vi "decodeModbusMessage.vi"(8 "error in (no error)":errorcluster, 10 "Enc_values_in":T1, 11 "VISA resource name":refnum<visa-resource-name>) -> (0 "error out":errorcluster, 2 "Enc_values_out 2":T1, 3 "VISA Refnum out":refnum<visa-resource-name>)   [LabVIEW 2026]
uses:
  Control/Ctr_Enc_Values.ctl
  Control/Ctrl_Motores_Valores.ctl
  Control/Ctrl_Errores.ctl
  Control/Ctrl_Modbus64.ctl
  Control/Ctrl_Datos6Motores.ctl
  Control/Ctrl_Modbus13.ctl
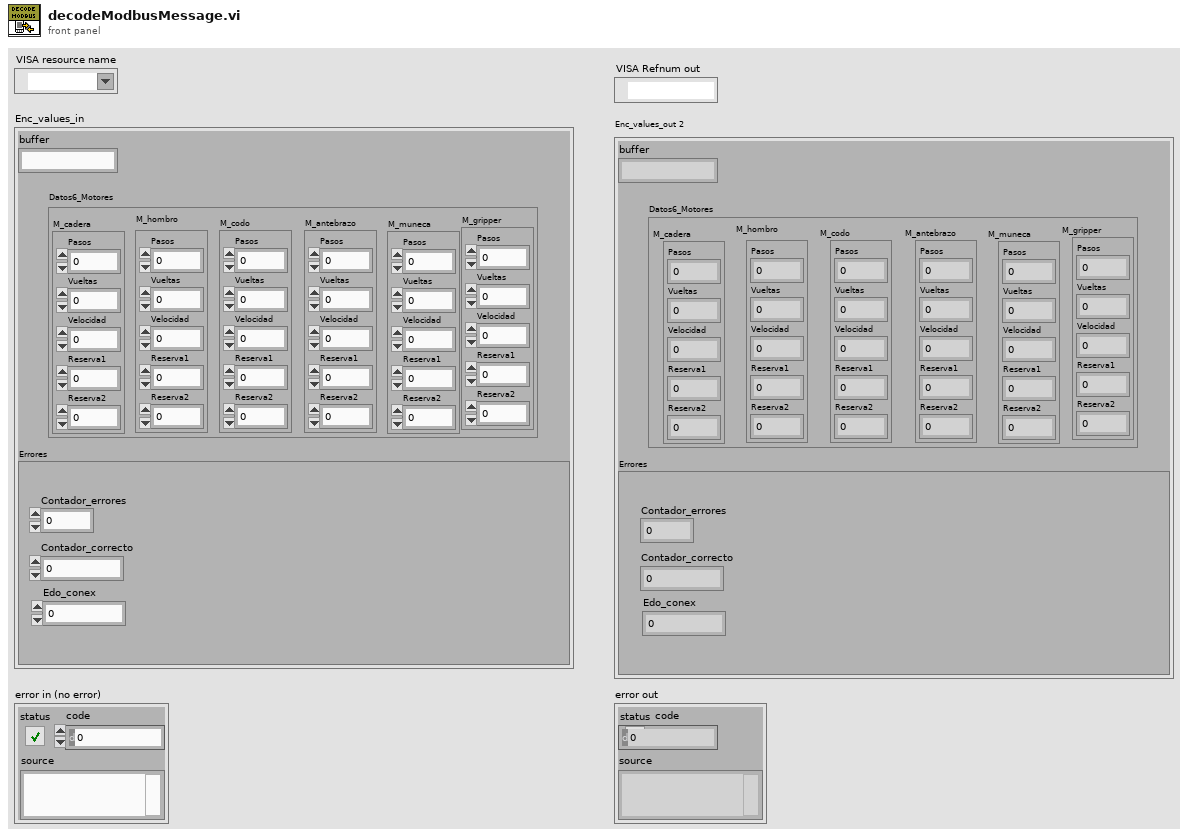
[diagram p1: front panel]
types:
  T1 = typedef "Ctr_Enc_Values.ctl" = cluster{"buffer":string, "Datos6_Motores":cluster{"M_cadera":T2, "M_hombro":T2, "M_codo":T2, "M_antebrazo":T2, "M_muneca":T2, "M_gripper":T2}, "Errores":T3}
  T2 = typedef "Ctrl_Motores_Valores.ctl" = cluster{"Pasos":i32, "Vueltas":i16, "Velocidad":i16, "Reserva1":u8, "Reserva2":u8}
  T3 = typedef "Ctrl_Errores.ctl" = cluster{"Contador_correcto":u32, "Contador_errores":u32, "Edo_conex":u32}
  T4 = typedef "Ctrl_Modbus64.ctl" = cluster{"header":u8, "fx":u8, "longitud":u8, "Datos6_Motores":T5, "checksum":u8}
  T5 = typedef "Ctrl_Datos6Motores.ctl" = cluster{"M_cadera":T2, "M_hombro":T2, "M_codo":T2, "M_antebrazo":T2, "M_muneca":T2, "M_gripper":T2}
  T6 = enum16{"big-endian, network order", "native, host order", "little-endian"}
  T7 = typedef "Ctrl_Modbus13.ctl" = cluster{"header":u8, "funcion":u8, "longitud":u8, "identificador":u8, "M_individual":T2, "checksum":u8}
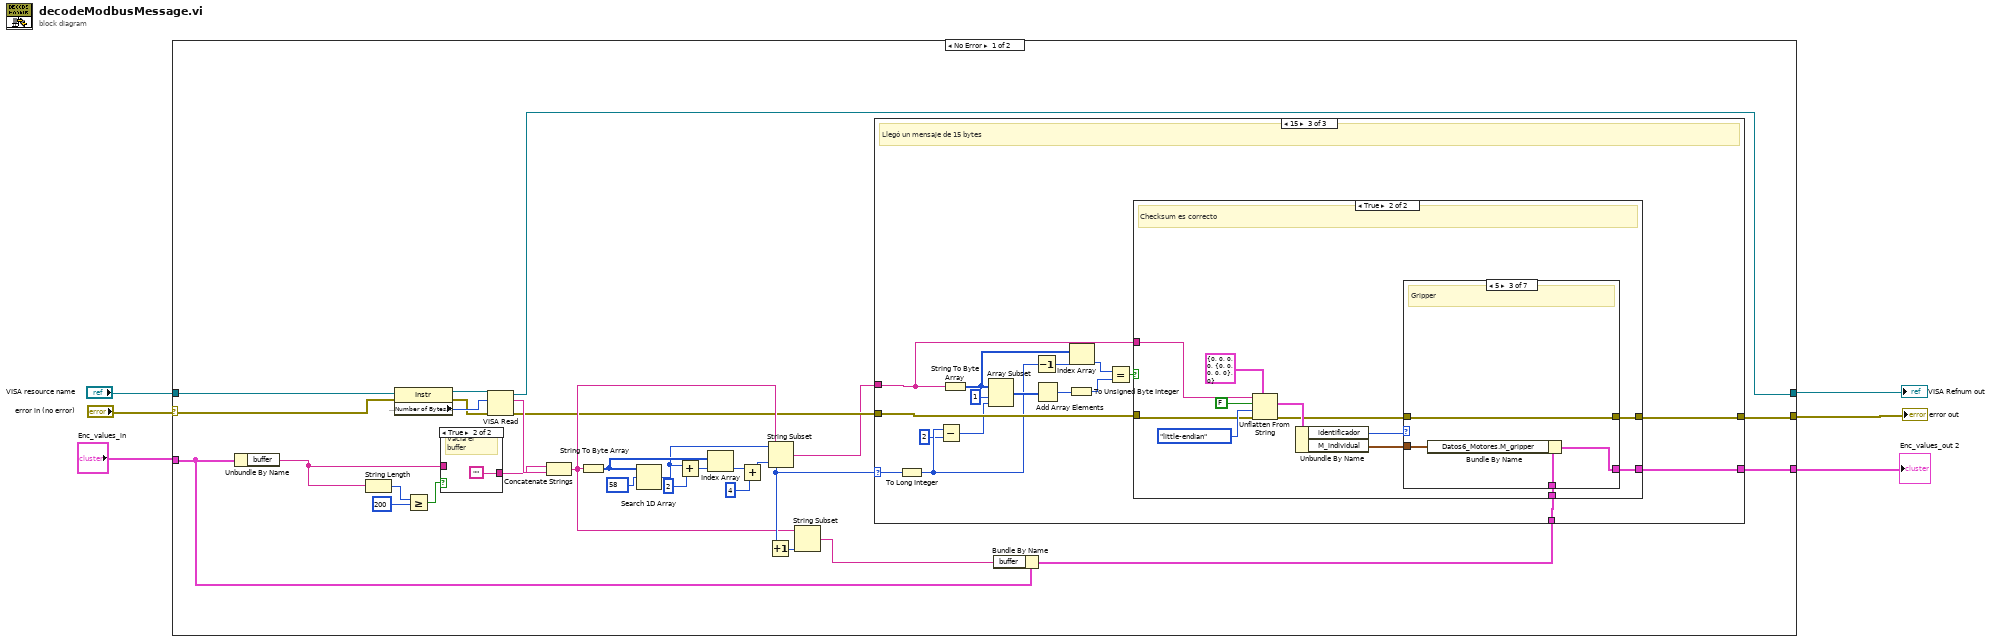
[diagram p0: block diagram]
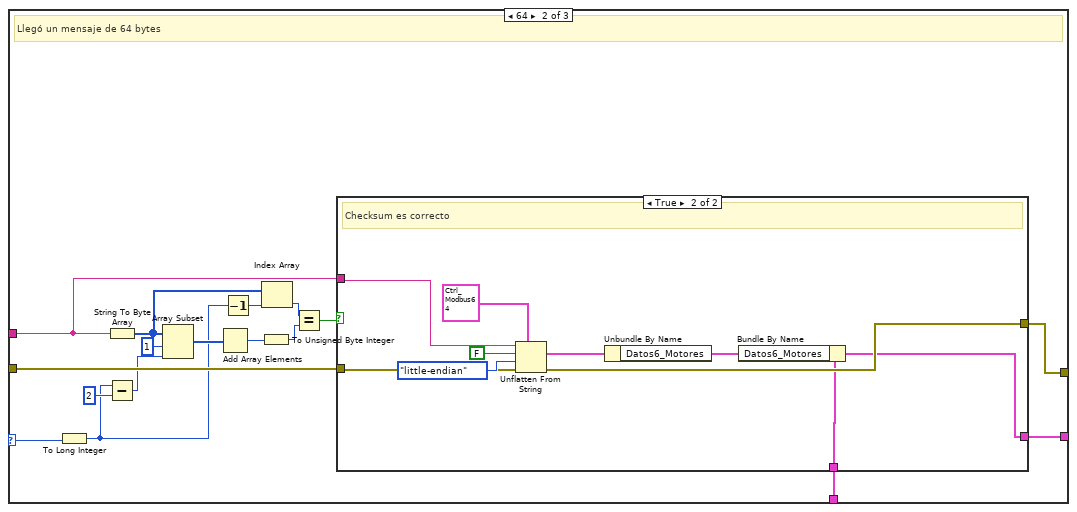
[diagram p4: hidden frame]
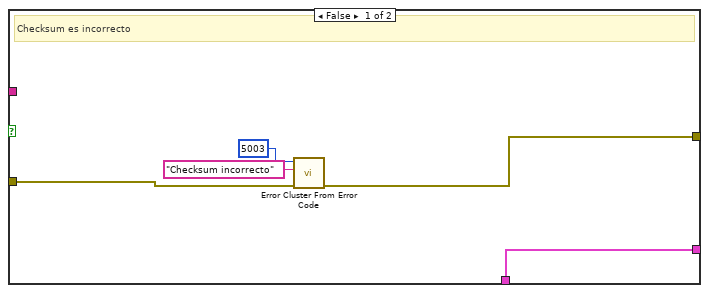
[diagram p5: hidden frame]
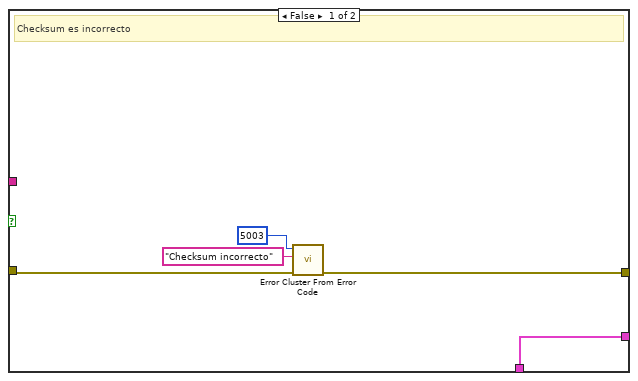
[diagram p6: hidden frame]
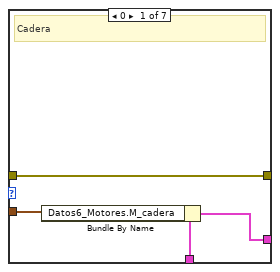
[diagram p7: hidden frame]
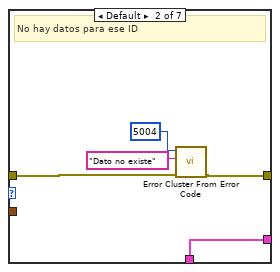
[diagram p8: hidden frame]
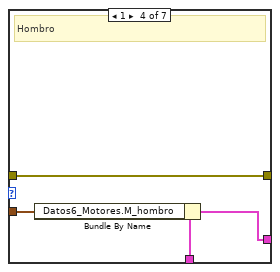
[diagram p9: hidden frame]
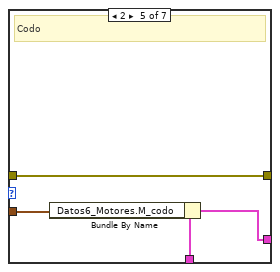
[diagram p10: hidden frame]
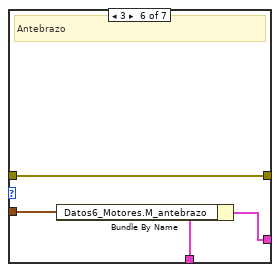
[diagram p11: hidden frame]
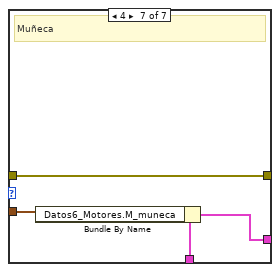
[diagram p12: hidden frame]
diagram:
  n1 = case shown="No Error" "error in (no error)" {
    selector: "error in (no error)" -> [w34 w137]
    tunnel: [w17 w137] -> w5
    tunnel: "VISA resource name" -> [w35 w136]
    tunnel: [w16 w136] -> w3
    tunnel: "Enc_values_in" -> [w9 w135]
    tunnel: [w7 w135] -> w1
    frame No Error {
      n2 = Unbundle By Name(w9) -> ("buffer"=w11:string)
      n3 = String Length(string=w11) -> (length=w15:i32)
      n4 = property class="Instr"(reference=w35, error in=w34) -> (reference out=w31:refnum<visa-resource-name>, error out=w32:errorcluster, "Serial Settings:Number of Bytes at Serial Port"=w33:u32)
      n5 = Greater Or Equal?(x=w15, y=200) -> (x >= y?=w13:bool)
      n6 = case shown="True" w13 {
        tunnel: [w36 ""] -> w12
        tunnel: w11 -> [w36 _]
        frame False {
        }
        frame True {
          # "Vacía el buffer"
        }
      }
      n7 = VISA Read(VISA resource name=w31, byte count=w33, error in (no error)=w32) -> (VISA resource name out=w16:refnum<visa-resource-name>, read buffer=w26:string, error out=w19:errorcluster)  [unwired: 1 out]
      n8 = Concatenate Strings(w12, w26) -> (w20:string)
      n9 = String To Byte Array(string=w20) -> (unsigned byte array=w29:u8[])
      n10 = Search 1D Array(1D array=w29, element=u8 58 ("y")) -> (index of element=w25:i32)  [unwired: 1 in]
      n11 = Add(x=w25, y=2) -> (x+y=w28:i32)
      n12 = Index Array(array=w29, index=w28) -> (element=w24:u8)
      n13 = Add(x=w24, y=u8 4) -> (x+y=w21:u8)
      n14 = Increment(x=w21) -> (x+1=w22:u8)
      n15 = String Subset(string=w20, offset (0)=w25, length (rest)=w21) -> (substring=w18:string)
      n16 = String Subset(string=w20, offset (0)=w22) -> (substring=w10:string)  [unwired: 1 in]
      n17 = Bundle By Name(cluster=w9, "buffer"=w10) -> (w8:T1)
      n18 = case shown="15" w21 {
        selector: w21 -> [_ w45 w77]
        tunnel: w18 -> [_ w47 w80]
        tunnel: w19 -> [w39 w49 w81]
        tunnel: [w39 w48 w79] -> w17
        tunnel: w8 -> [w38 w41 w73]
        tunnel: [w38 w40 w72] -> w7
        frame 0, Default {
          # "Mensaje vacío"
        }
        frame 64 {
          # "Llegó un mensaje de 64 bytes"
          n19 = To Long Integer(number=w45) -> (32bit integer=w42:i32)
          n20 = String To Byte Array(string=w47) -> (unsigned byte array=w53:u8[])
          n21 = Subtract(x=w42, y=2) -> (x-y=w44:i32)
          n22 = Array Subset(array=w53, index=1, length=w44) -> (w55:u8[])
          n23 = Add Array Elements(numeric array=w55) -> (sum=w54:u8)
          n24 = Decrement(x=w42) -> (x-1=w43:i32)
          n25 = To Unsigned Byte Integer(number=w54) -> (unsigned 8bit integer=w51:u8)
          n26 = Index Array(array=w53, index=w43) -> (element=w52:u8)
          n27 = Equal?(x=w52, y=w51) -> (x = y?=w50:bool)
          n28 = case shown="True" w50 {
            tunnel: w49 -> [w58 w69]
            tunnel: [w59 w68] -> w48
            tunnel: w47 -> [_ w67]
            tunnel: w41 -> [w57 w64]
            tunnel: [w57 w63] -> w40
            frame False {
              # "Checksum es incorrecto"
              n29 = call <vilib>:"Error Cluster From Error Code.vi"("error in (no error)"=w58, "error message (\"\")"="Checksum incorrecto" ("error message (\"\")"), "error code (0)"=5003) -> ("error out"=w59:errorcluster)  [unwired: 6 in]
            }
            frame True {
              # "Checksum es correcto"
              n30 = Unflatten From String(type=T4 {"header"=0, "fx"=0, "longitud"=0, "Datos6_Motores"={"M_cadera"={"Pasos"=0, "Vueltas"=0, "Velocidad"=0, "Reserva1"=0, "Reserva2"=0}, "M_hombro"={"Pasos"=0, "Vueltas"=0, "Velocidad"=0, "Reserva1"=0, "Reserva2"=0}, "M_codo"={"Pasos"=0, "Vueltas"=0, "Velocidad"=0, "Reserva1"=0, "Reserva2"=0}, "M_antebrazo"={"Pasos"=0, "Vueltas"=0, "Velocidad"=0, "Reserva1"=0, "Reserva2"=0}, "M_muneca"={"Pasos"=0, "Vueltas"=0, "Velocidad"=0, "Reserva1"=0, "Reserva2"=0}, "M_gripper"={"Pasos"=0, "Vueltas"=0, "Velocidad"=0, "Reserva1"=0, "Reserva2"=0}}, "checksum"=0} ("modbus_64"), binary string=w67, data includes array or string size? (T)=FALSE, byte order (0:big-endian, network order)=T6."little-endian", error in (no error)=w69) -> (value=w66:T4, error out=w68:errorcluster)  [unwired: 1 out]
              n31 = Unbundle By Name(w66) -> ("Datos6_Motores"=w62:T5)
              n32 = Bundle By Name(cluster=w64, "Datos6_Motores"=w62) -> (w63:T1)
            }
          }
        }
        frame 15 {
          # "Llegó un mensaje de 15 bytes"
          n33 = To Long Integer(number=w77) -> (32bit integer=w75:i32)
          n34 = Subtract(x=w75, y=2) -> (x-y=w76:i32)
          n35 = String To Byte Array(string=w80) -> (unsigned byte array=w85:u8[])
          n36 = Array Subset(array=w85, index=1, length=w76) -> (w87:u8[])
          n37 = Decrement(x=w75) -> (x-1=w78:i32)
          n38 = Add Array Elements(numeric array=w87) -> (sum=w86:u8)
          n39 = To Unsigned Byte Integer(number=w86) -> (unsigned 8bit integer=w83:u8)
          n40 = Index Array(array=w85, index=w78) -> (element=w84:u8)
          n41 = Equal?(x=w84, y=w83) -> (x = y?=w82:bool)
          n42 = case shown="True" w82 {
            tunnel: w81 -> [w90 w103]
            tunnel: w80 -> [_ w102]
            tunnel: [w89 w99] -> w72
            tunnel: [w91 w98] -> w79
            tunnel: w73 -> [w89 w95]
            frame False {
              # "Checksum es incorrecto"
              n43 = call <vilib>:"Error Cluster From Error Code.vi"("error in (no error)"=w90, "error message (\"\")"="Checksum incorrecto" ("error message (\"\")"), "error code (0)"=5003) -> ("error out"=w91:errorcluster)  [unwired: 6 in]
            }
            frame True {
              # "Checksum es correcto"
              n44 = Unflatten From String(type=T7 {"header"=0, "funcion"=0, "longitud"=0, "identificador"=0, "M_individual"={"Pasos"=0, "Vueltas"=0, "Velocidad"=0, "Reserva1"=0, "Reserva2"=0}, "checksum"=0} ("Modbus_13b"), binary string=w102, data includes array or string size? (T)=FALSE, byte order (0:big-endian, network order)=T6."little-endian", error in (no error)=w103) -> (value=w101:T7, error out=w97:errorcluster)  [unwired: 1 out]
              n45 = Unbundle By Name(w101) -> ("identificador"=w100:u8, "M_individual"=w94:T2)
              n46 = case shown="5" w100 {
                tunnel: [w107 w114 w115 w122 w125 w128 w132] -> w99
                tunnel: [w109 w110 w118 w121 w126 w130 w134] -> w98
                tunnel: w97 -> [w109 w111 w118 w121 w126 w130 w134]
                tunnel: w95 -> [w108 w114 w116 w120 w124 w129 w133]
                tunnel: w94 -> [w106 _ w117 w119 w123 w127 w131]
                frame 0 {
                  # "Cadera"
                  n47 = Bundle By Name(cluster=w108, "Datos6_Motores.M_cadera"=w106) -> (w107:T1)
                }
                frame Default {
                  # "No hay datos para ese ID"
                  n48 = call <vilib>:"Error Cluster From Error Code.vi"("error in (no error)"=w111, "error message (\"\")"="Dato no existe" ("error message (\"\")"), "error code (0)"=5004) -> ("error out"=w110:errorcluster)  [unwired: 6 in]
                }
                frame 5 {
                  # "Gripper"
                  n49 = Bundle By Name(cluster=w116, "Datos6_Motores.M_gripper"=w117) -> (w115:T1)
                }
                frame 1 {
                  # "Hombro"
                  n50 = Bundle By Name(cluster=w120, "Datos6_Motores.M_hombro"=w119) -> (w122:T1)
                }
                frame 2 {
                  # "Codo"
                  n51 = Bundle By Name(cluster=w124, "Datos6_Motores.M_codo"=w123) -> (w125:T1)
                }
                frame 3 {
                  # "Antebrazo"
                  n52 = Bundle By Name(cluster=w129, "Datos6_Motores.M_antebrazo"=w127) -> (w128:T1)
                }
                frame 4 {
                  # "Muñeca"
                  n53 = Bundle By Name(cluster=w133, "Datos6_Motores.M_muneca"=w131) -> (w132:T1)
                }
              }
            }
          }
        }
      }
    }
    frame Error {
    }
  }
  "VISA Refnum out" <- w3
  "error out" <- w5
  "Enc_values_out 2" <- w1
